vi "Launch Login Process.vi"(8 "error in (no error)":errorcluster, 11 "TopLevel in":refnum<class "TopLevel.lvclass">) -> (0 "error out":errorcluster, 3 "TopLevel out":refnum<class "TopLevel.lvclass">)   [LabVIEW 2022 SP3, in "TopLevel.lvclass"]
uses:
  TopLevel.lvclass
  Login_Process.vi
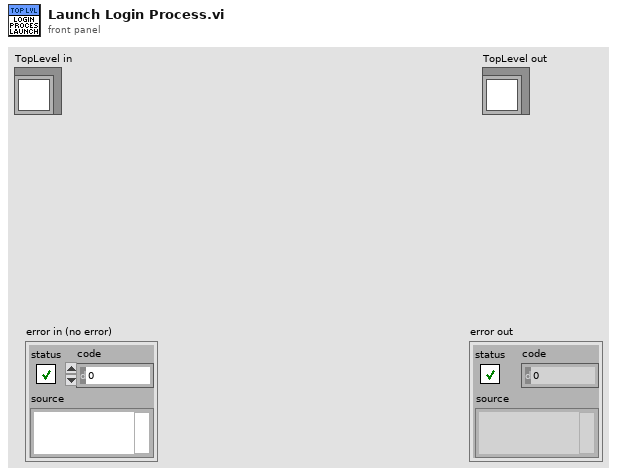
[diagram p1: front panel]
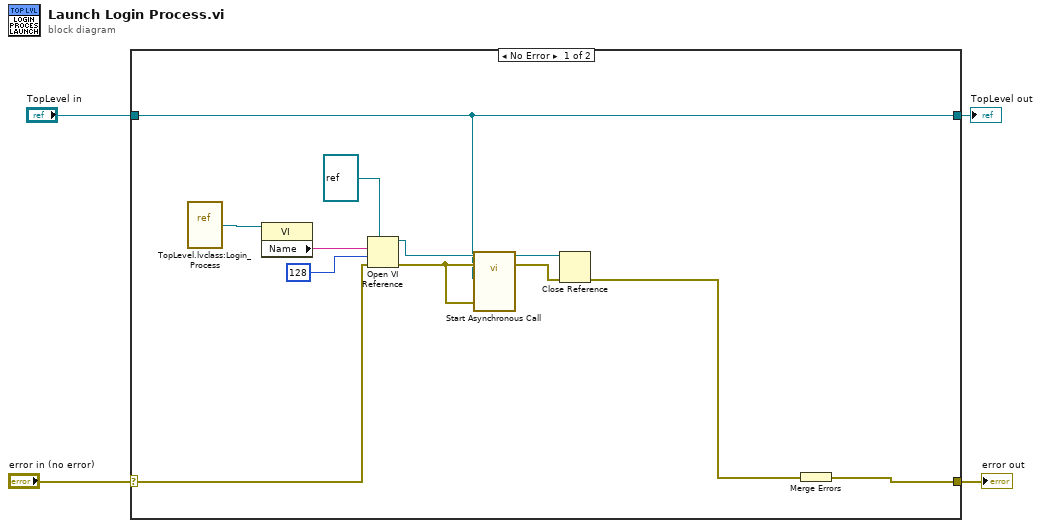
[diagram p0: block diagram]
diagram:
  n1 = case shown="No Error" "error in (no error)" {
    selector: "error in (no error)" -> [w12 w18]
    tunnel: [w7 w18] -> w3
    tunnel: "TopLevel in" -> [w5 w17]
    tunnel: [w5 w17] -> w1
    frame No Error {
      n2 = vi-ref "TopLevel.lvclass:Login_Process.vi"() -> (w16:refnum<vi>)
      n3 = property class="VI"(reference=w16) -> ("Name"=w15:string)  [unwired: 1 in, 2 out]
      n4 = Open VI Reference(type specifier VI Refnum (for type only)=refnum<vi> refnum, vi path=w15, options=128, error in (no error)=w12) -> (vi reference=w11:refnum<vi>, error out=w10:errorcluster)  [unwired: 2 in]
      n5 = call-by-ref "Start Asynchronous Call"(reference=w11, error in=w10, 8:"error in (no error)"=w10, "TopLevel in"=w5) -> (reference out=w9:refnum<vi>, error out=w8:errorcluster)  [unwired: 8 in, 2 out]
      n6 = Close Reference(reference=w9, error in (no error)=w8) -> (error out=w6:errorcluster)
      n7 = Merge Errors(w6) -> (w7:errorcluster)
    }
    frame Error {
    }
  }
  "error out" <- w3
  "TopLevel out" <- w1
